vi "PH_Img_BaseClass.evt Call set Timeout.vi"(0 "i ref in":refnum<vi>, 1 "Instance":string, 3 "Timeout [ms]":i32, 5 "error in (no error)":errorcluster) -> (14 "i ref out":refnum<vi>, 19 "error out":errorcluster)   [LabVIEW 2014, in "PH_Img_BaseClass.lvlib"]
doc: "This VI calls the event case \"SetTO\" by a simple call."
uses:
  PH_Img_BaseClass.lvlib
  CS_Core/CSSystem/CoreLib/CoreLib.int 2 byte array.vi
  CS_Core/CSSystem/CoreLib/CoreLib.lvlib
  CS_Core/BaseProcess/BaseProcess.lvlib
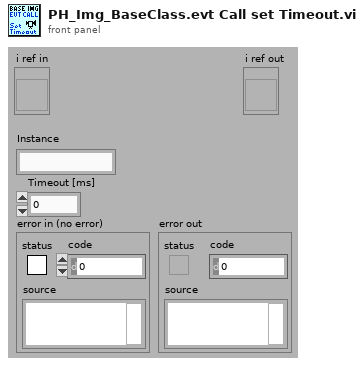
[diagram p1: front panel]
types:
  T1 = typedef "CoreDefs.rawDataType.ctl" = i8[]
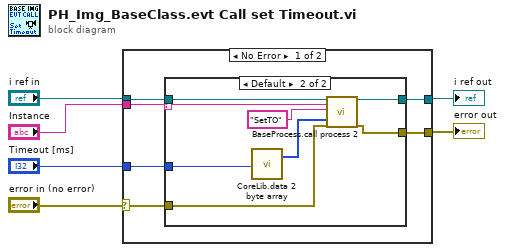
[diagram p0: block diagram]
diagram:
  n1 = case shown="No Error" "error in (no error)" {
    selector: "error in (no error)" -> [w9 w23]
    tunnel: [w12 w24] -> w3
    tunnel: [w11 w23] -> w2
    tunnel: "i ref in" -> [w10 w24]
    tunnel: "Instance" -> [w8 _]
    tunnel: "Timeout [ms]" -> [w7 _]
    frame No Error {
      n2 = case shown="Default" w8 {
        selector: w8 -> [_ w15]
        tunnel: [w14 w21] -> w12
        tunnel: [w13 w20] -> w11
        tunnel: w10 -> [w14 w19]
        tunnel: w9 -> [w13 w17]
        tunnel: w7 -> [_ w16]
        frame "N/A" {
        }
        frame Default {
          n3 = call-poly "CoreLib.data 2 byte array.vi"("i32"=w16) -> ("byteArray out"=w18:T1)  [unwired: 18 in]
          n4 = call "BaseProcess.call process 2.vi"("i ref in"=w19, "Object"=w15, "Selector"="SetTO", "Data"=w18, "error in (no error)"=w17) -> ("i ref out"=w21:refnum<vi>, "error out"=w20:errorcluster)  [unwired: 13 in]
        }
      }
    }
    frame Error {
    }
  }
  "i ref out" <- w3
  "error out" <- w2
